vi "List Files By Timestamp.vi"(8 "error in (no error)":errorcluster, 9 "Ascending? (F)":bool, 10 "Pattern (\"\")":string, 11 "Path":path) -> (0 "error out":errorcluster, 2 "Standard Output":string, 3 "File Names":string[](array[string]))   [LabVIEW 2011]
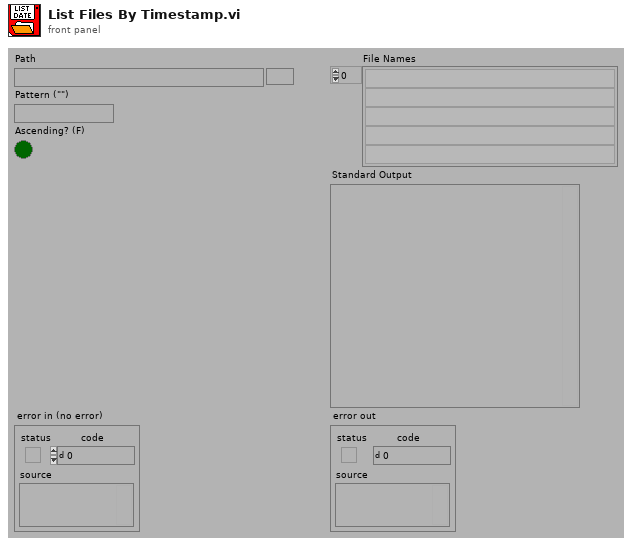
[diagram p1: front panel]
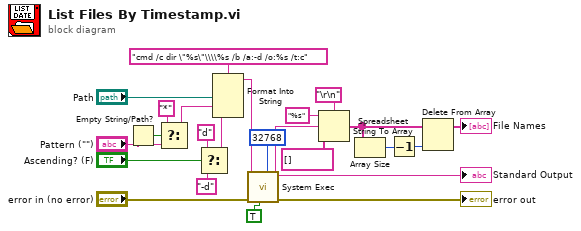
[diagram p0: block diagram]
diagram:
  n1 = Empty String/Path?(string/path="Pattern (\"\")") -> (empty?=w11:bool)
  n2 = Select(t="*", s=w11, f="Pattern (\"\")") -> (s? t:f=w3:string)
  n3 = Select(t="d", s="Ascending? (F)", f="-d" ("t")) -> (s? t:f=w2:string)
  n4 = Format Into String(format string="cmd /c dir \"%s\"\\\\%s /b /a:-d /o:%s /t:c" ("command line"), "Path", w3, w2) -> (resulting string=w15:string)  [unwired: 2 in, 1 out]
  n5 = call <vilib>:"System Exec.vi"("expected output size  (4096)"=u32 32768, "run minimized? (F)"=TRUE, "error in (no error)"="error in (no error)", "command line"=w15) -> ("error out"=→"error out":errorcluster, "standard output"=w22:string)  [unwired: 3 in, 3 out]
  "Standard Output" <- w22
  n6 = Spreadsheet String To Array(delimiter (Tab)="\r\n", format string="%s", spreadsheet string=w22, array type (2D Dbl)=string[] []) -> (array=w13:string[])
  n7 = Array Size(array=w13) -> (size(s)=w14:i32)
  n8 = Decrement(x=w14) -> (x-1=w8:i32)
  n9 = Delete From Array(array=w13, index=w8) -> (array with subset deleted=→"File Names":string[])  [unwired: 1 in, 1 out]
